vi "StopButton.vi"() -> ()   [LabVIEW 2015, in "ECS-RT.lvlib"]
uses:
  ECS-RT.lvlib
panel:
  in  "Stop Button":bool
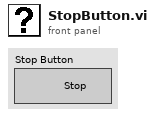
[diagram p1: front panel]
diagram:
